vi "HoloPy_template.vi"() -> ()   [LabVIEW 2023, in "holoTracker.lvlib"]
uses:
  holoTracker.lvlib
  subVis/HologramInfo.ctl
  subVis/analyse_parameters.ctl
  CCL_parameters.ctl
panel:
  in  "analyse parameters":T1={"propagation"={"distance ini"=0.0, "number of planes"=0, "step"=0.0, "Fourier BP filter (pix)"={"High pass (0=none)"=0.0, "Low Pass (0=none)"=0.0}}, "Focus"={"Type"=enum."SUM_OF_INTENSITY", "Sum size"=1}, "Remove mean Hologram"=FALSE, "CCL parameters"={"Threshold ( N x Standard deviation)"=10.0, "Connectivity"=enum."6", "min voxel"=1.0, "max voxel"=1.0}} {"CCL parameters"."max voxel" min=0.0 max=0.0; "CCL parameters"."min voxel" min=1.0 max=100.0; "CCL parameters"."Threshold ( N x Standard deviation)" min=1.0 max=100.0; "Focus"."Sum size" min=1 max=100; "propagation"."Fourier BP filter (pix)"."Low Pass (0=none)" format="%#_6e"; "propagation"."step" format="%#_6e"; "propagation"."distance ini" format="%#_6e"}
  in  "HOLO INFO":T3 {"Holo size X" format="%#_6e"; "wavelength" format="%#_6e"}
  out "return value":string
  in  "Refnum in":refnum<k35>
  out "Refnum out":refnum<k35>
  in  "error in (no error)":errorcluster
  out "error out":errorcluster
  in  "Application Directory":path
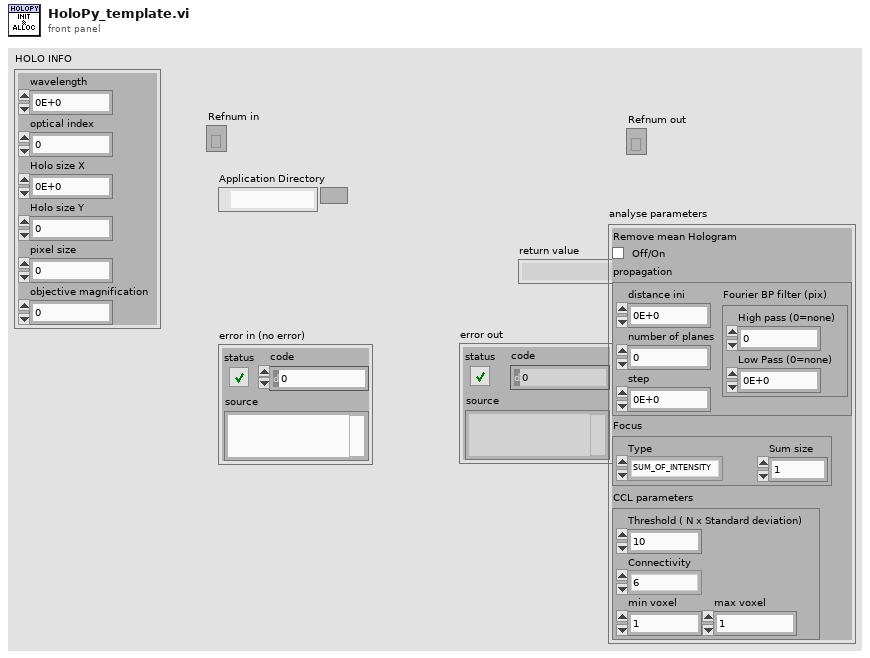
[diagram p1: front panel]
types:
  T1 = typedef "holoTracker.lvlib/analyse_parameters.ctl" = cluster{"propagation":cluster{"distance ini":dbl, "number of planes":i32, "step":dbl, "Fourier BP filter (pix)":cluster{"High pass (0=none)":dbl, "Low Pass (0=none)":dbl}}, "Focus":cluster{"Type":enum16{"SUM_OF_INTENSITY", "SUM_OF_LAPLACIAN", "SUM_OF_VARIANCE", "TENENGRAD"}, "Sum size":i32}, "Remove mean Hologram":bool, "CCL parameters":T2}
  T2 = typedef "CCL_parameters.ctl" = cluster{"Threshold ( N x Standard deviation)":dbl, "Connectivity":enum16{"6", "18", "26"}, "min voxel":dbl, "max voxel":dbl}
  T3 = typedef "holoTracker.lvlib/HologramInfo.ctl" = cluster{"wavelength":sgl, "optical index":sgl, "Holo size X":i32, "Holo size Y":i32, "pixel size":sgl, "objective magnification":sgl}
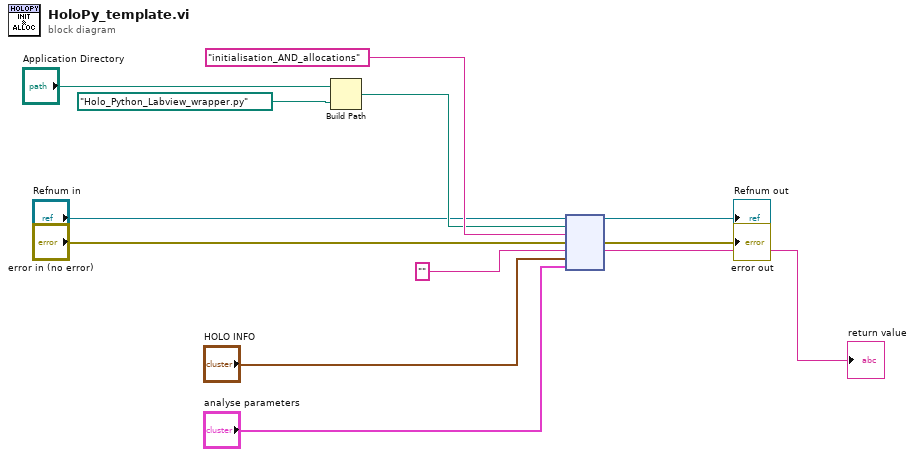
[diagram p0: block diagram]
diagram:
  n1 = Build Path(base path="Application Directory", name or relative path=path "Holo_Python_Labview_wrapper.py") -> (appended path=w11:path)
  n2 = node("Refnum in", w11, "initialisation_AND_allocations" ("function name"), "error in (no error)", "", "HOLO INFO", "analyse parameters") -> (→"Refnum out":refnum<k35>, →"error out":errorcluster, →"return value":string)  [unwired: 2 in, 2 out]
